vi "T7MOD_Read_INT32_Register.vi"(8 "error in":errorcluster, 9 "LabJack INT32 Register":i32=55122, 10 "Remote Port":u16=502, 11 "Remote IP Address":string="192.168.1.15") -> (0 "error out":errorcluster, 1 "Read At":timestamp, 2 "Raw Data Read":u16[](array[numeric]), 3 "Read INT32":i32)   [LabVIEW 2018]
panel:
  # "Output"
  # "TCP Parameters"
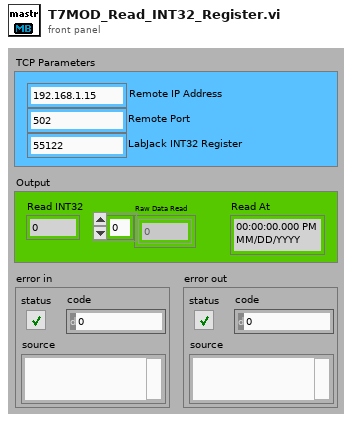
[diagram p1: front panel]
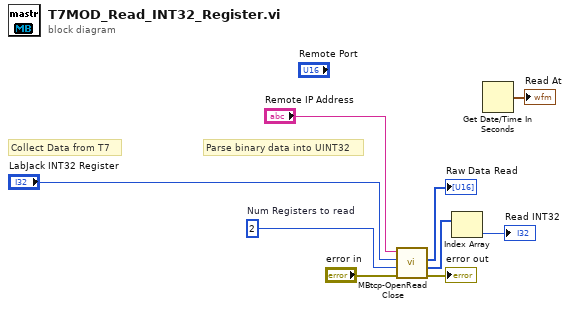
[diagram p0: block diagram]
diagram:
  w6 = 2  # Num Registers to read
  # "Parse binary data into UINT32"
  # "Collect Data from T7"
  n1 = call "MBtcp-OpenReadClose.vi"("error in (no error)"="error in", "nRegisters"=w6, "RegisterAddr"="LabJack INT32 Register", "IP Address(:port)"="Remote IP Address") -> ("error out"=→"error out":errorcluster, "32bitValues"=w3:u32[], "16bitValues"=→"Raw Data Read":u16[])  [unwired: 5 in]
  n2 = Index Array(array=w3) -> (element=→"Read INT32":u32)  [unwired: 1 in]
  n3 = Get Date/Time In Seconds() -> (seconds since 1Jan1904=→"Read At":timestamp)
